vi "Read TCP FIFO.vi"(6 "Error In":errorcluster, 9 "Vessel.lvclass":refnum<class "Vessel.lvclass">) -> (0 "Error Out":errorcluster, 3 "Vessel.lvclass 2":refnum<class "Vessel.lvclass">)   [LabVIEW 2014, in "Vessel.lvclass"]
uses:
  Vessel.lvclass
  Vessel.lvclass/Vessel.ctl
  Supervisor/Supervisor.lvclass
panel:
  out "UDP GPS":string
  out "UDP APOS":string
  out "Camera Trigger Message":string
  out "UDP error out":errorcluster
  out "APOS NED":dbl[](array[numeric]) format="%#.3f"
  out "kPa":dbl=100000.0 format="%#.1f"
  in  "depth ring":u16(ring)=2 items=["Saiv", "DVL", "Digiquartz"]
  out "DVL":string
  out "MT_BITS":u8[](array[numeric])
  out "Pos_s":dbl[](array[numeric])
  out "Altitudes":dbl[](array[numeric])
  out "Telebuf":u8[](array[numeric])
  out "NAVI OK":string
  out "MT_DATA":sgl[](array[numeric])
  in  "alt off [m]":dbl=0.2
  out "dvl_m":dbl[](array[numeric])
  out "MRU out":dbl[](array[numeric])
  out "Signals out":dbl[](array[numeric]) format="%#.2f"
  # "10."
  # "20."
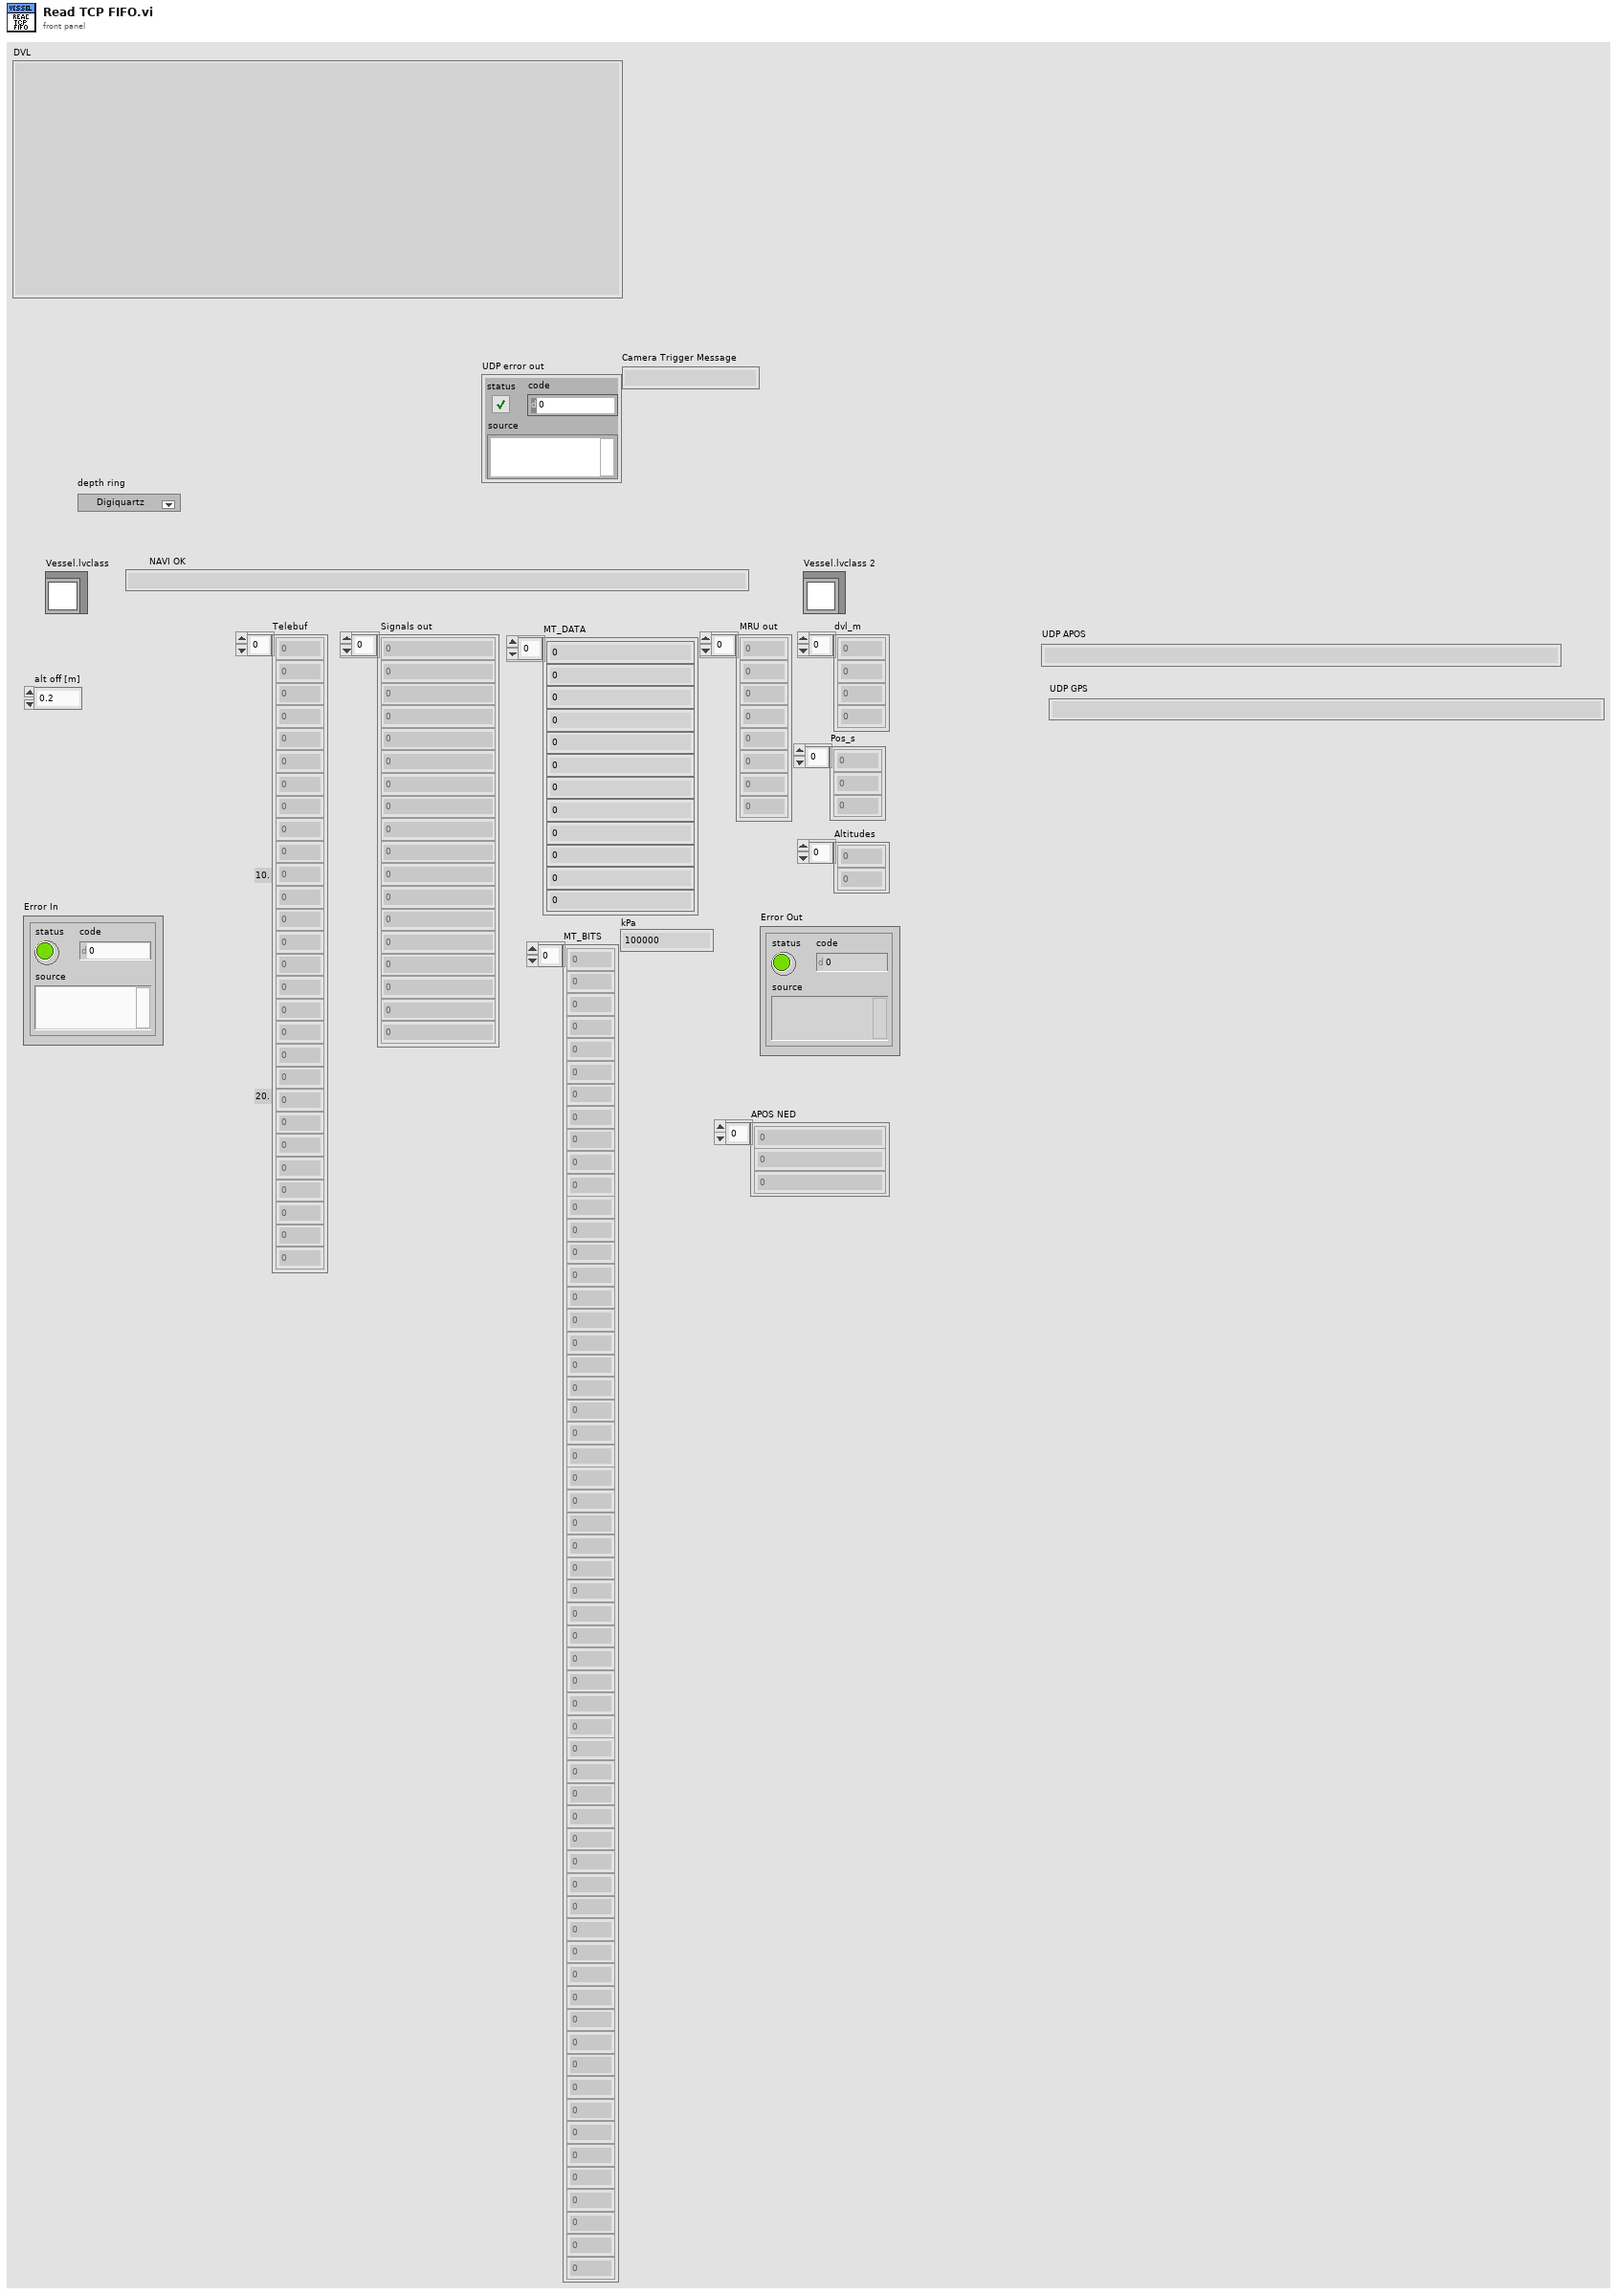
[diagram p1: front panel]
types:
  T1 = cluster{"Axis Translation":cluster{"X-Axis":dbl, "Y-Axis":dbl, "Z-Axis":dbl}, "Axis Rotation":cluster{"X-Axis":dbl, "Y-Axis":dbl, "Z-Axis":dbl}}
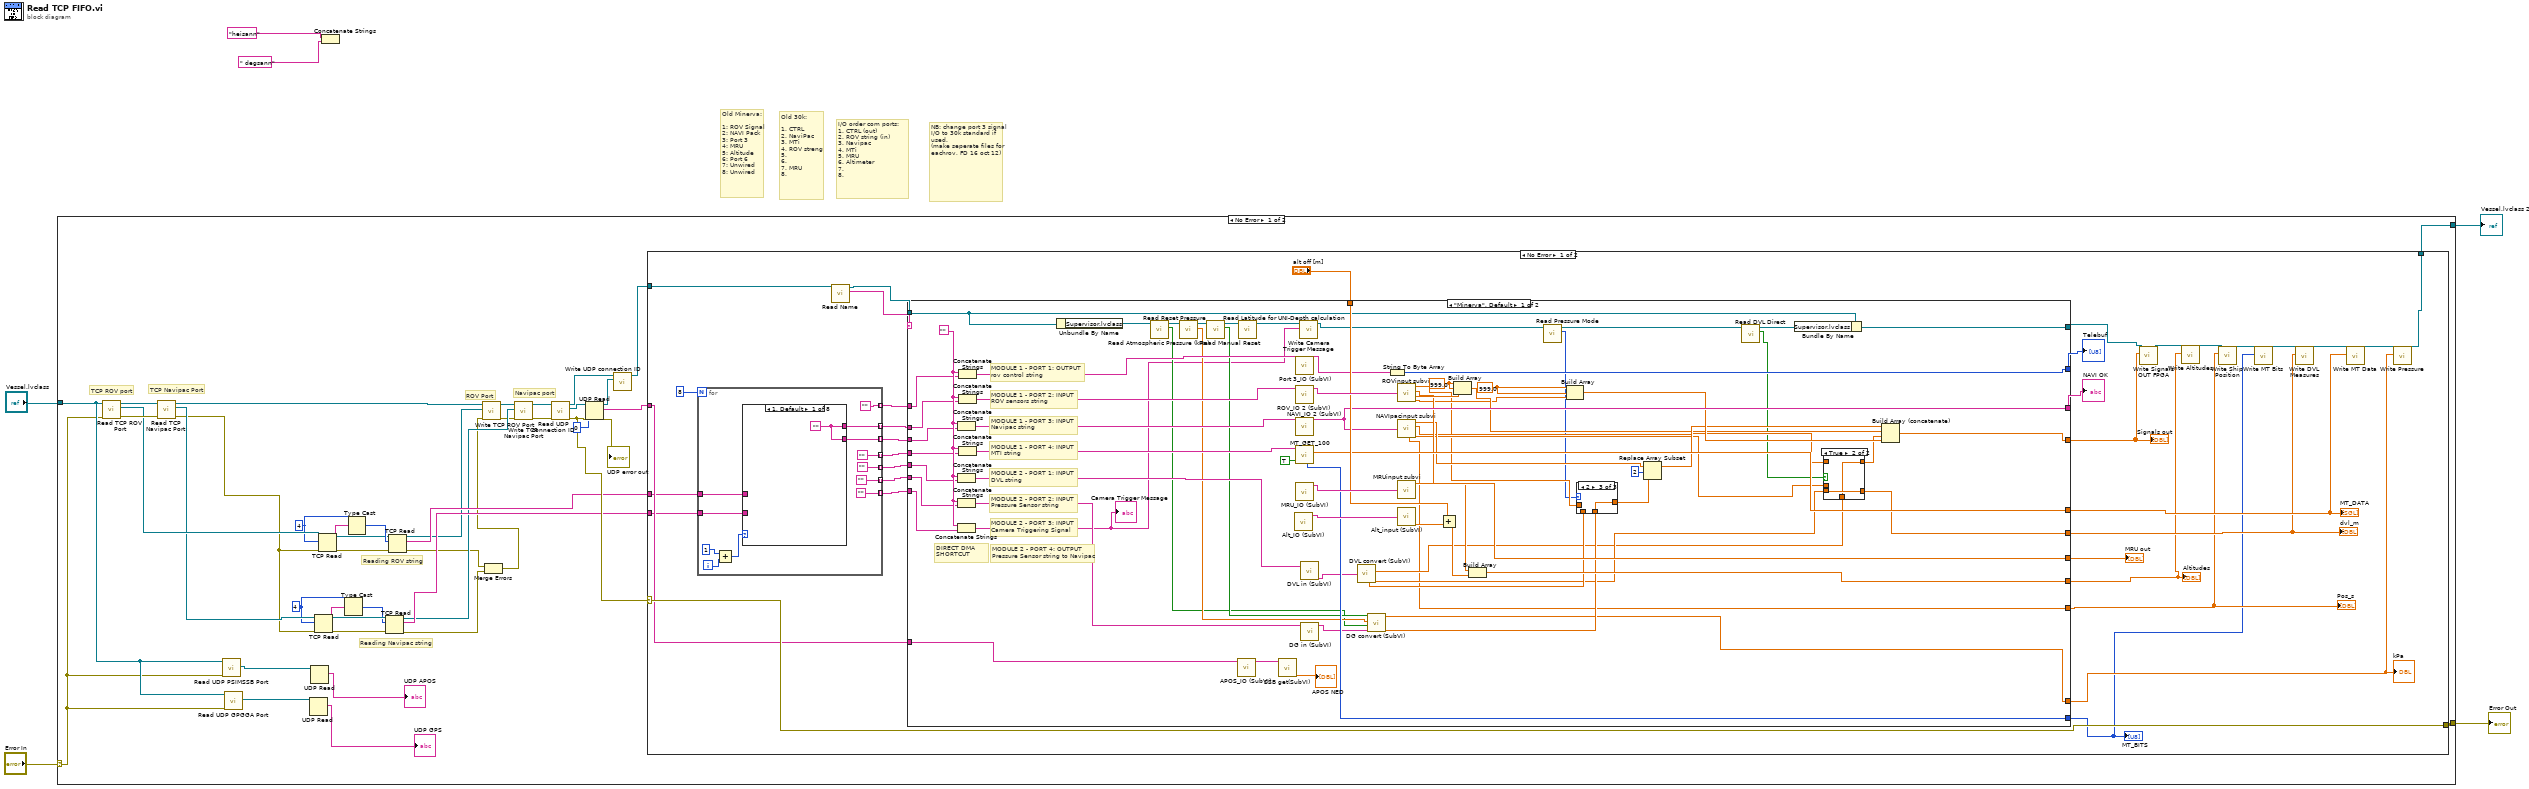
[diagram p0: block diagram]
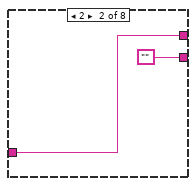
[diagram p2: hidden frame]
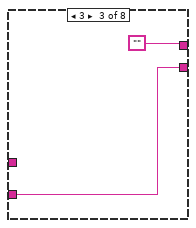
[diagram p3: hidden frame]
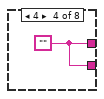
[diagram p4: hidden frame]
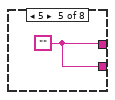
[diagram p5: hidden frame]
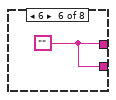
[diagram p6: hidden frame]
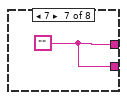
[diagram p7: hidden frame]
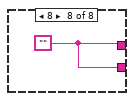
[diagram p8: hidden frame]
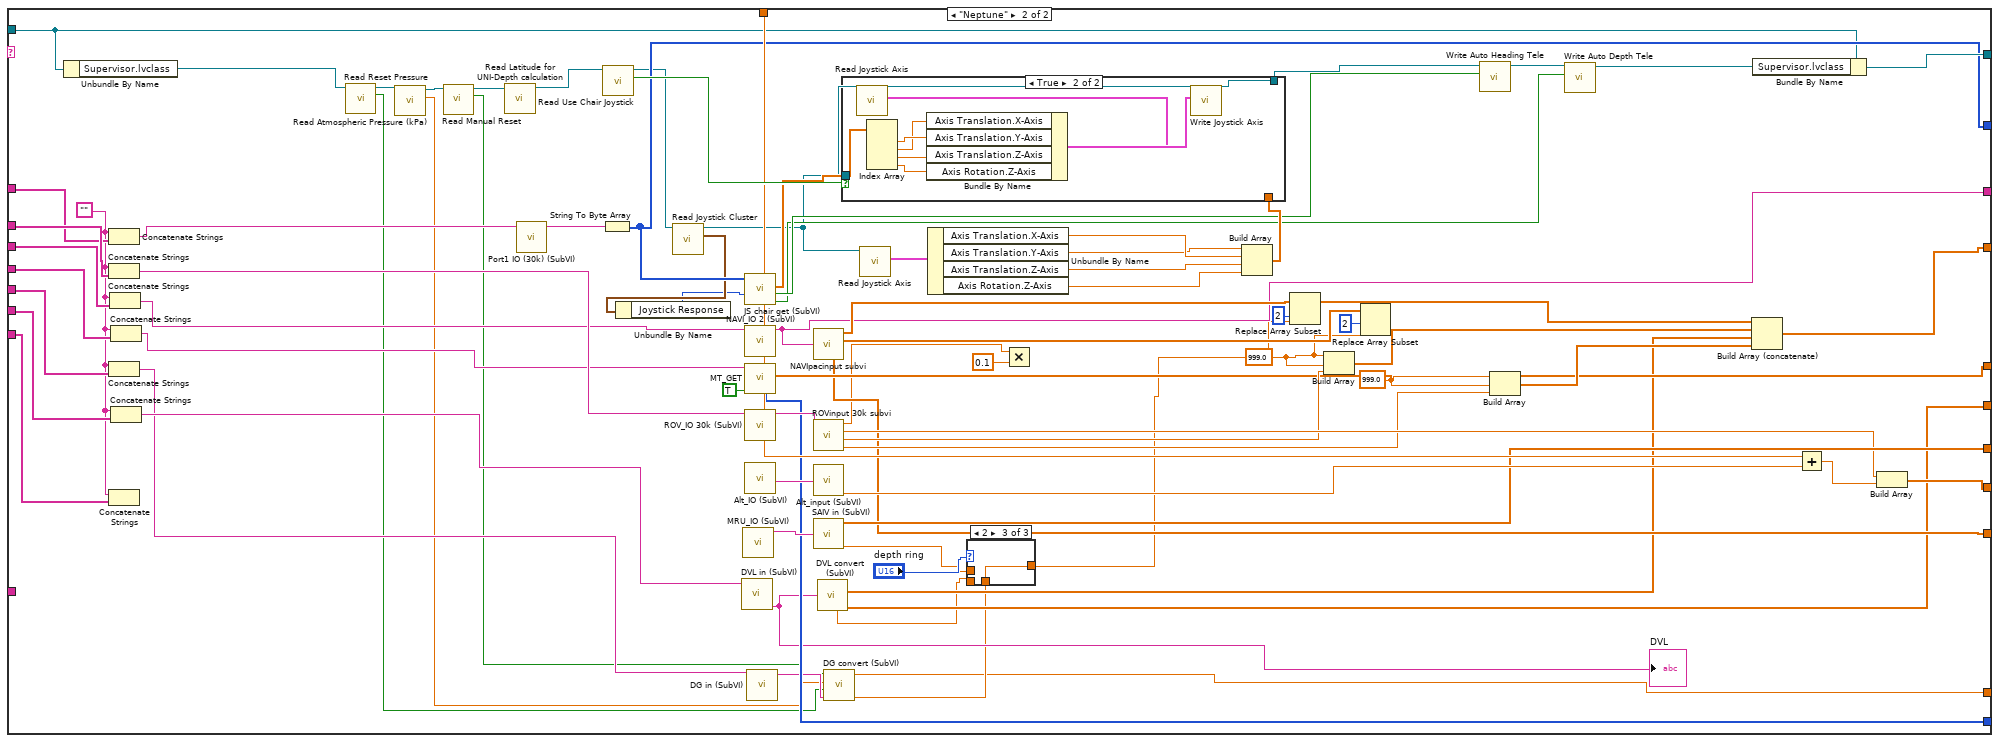
[diagram p12: hidden frame]
diagram:
  # "NB: change port 3 signal I/O to 30k standard if used. \n(make seperate files for eachrov, FD 16 oct 12)"
  # "I/O order com ports:\n1. CTRL (out)\n2. ROV string (in)\n3. Navipac\n4. MTi\n5. MRU\n6. Altimeter\n7. \n8."
  # "Old 30k:\n\n1. CTRL\n2. NaviPac\n3. MTi\n4. ROV streng\n5.\n6.\n7. MRU\n8."
  # "Old Minerva:\n\n1: ROV Signal\n2: NAVI Pack\n3: Port 3\n4: MRU\n5: Altitude \n6: Port 6\n7: Unwired\n8: Unwired"
  n1 = case shown="No Error" "Error In" {
    selector: "Error In" -> [w11 w282]
    tunnel: "Vessel.lvclass" -> [w12 w283]
    tunnel: [w49 w282] -> w4
    tunnel: [w48 w283] -> w3
    frame No Error {
      w19 = 4
      w20 = 4
      # "Reading ROV string"
      # "Reading Navipac string"
      # "Navipac port"
      # "ROV Port"
      # "TCP Navipac Port"
      # "TCP ROV port"
      n2 = call-dynamic "Read TCP ROV Port.vi"("error in (no error)"=w11, "Vessel in"=w12) -> ("error out"=w36:errorcluster, "TCP Network Connection Refnum"=w35:refnum<k5>, "Vessel out"=w37:refnum<class "Vessel.lvclass">)  [unwired: 7 in]
      n3 = call-dynamic "Read TCP Navipac Port.vi"("error in (no error)"=w36, "Vessel in"=w37) -> ("error out"=w33:errorcluster, "TCP Network Connection Refnum"=w34:refnum<k5>, "Vessel out"=w32:refnum<class "Vessel.lvclass">)  [unwired: 7 in]
      n4 = call-dynamic "Read UDP PSIMSSB Port.vi"("error in (no error)"=w11, "Vessel in"=w12) -> ("UDP Network Connection Refnum"=w10:refnum<k16>)  [unwired: 7 in, 2 out]
      n5 = call-dynamic "Read UDP GPGGA Port.vi"("error in (no error)"=w11, "Vessel in"=w12) -> ("UDP Network Connection Refnum"=w9:refnum<k16>)  [unwired: 7 in, 2 out]
      n6 = UDP Read(connection ID=w9) -> (data out=→"UDP GPS":string)  [unwired: 3 in, 4 out]
      n7 = UDP Read(connection ID=w10) -> (data out=→"UDP APOS":string)  [unwired: 3 in, 4 out]
      n8 = TCP Read(connection ID=w34, bytes to read=w20, error in (no error)=w33) -> (connection ID out=w24:refnum<k5>, data out=w22:string, error out=w23:errorcluster)  [unwired: 2 in]
      n9 = TCP Read(connection ID=w35, bytes to read=w19, error in (no error)=w33) -> (connection ID out=w15:refnum<k5>, data out=w17:string, error out=w16:errorcluster)  [unwired: 2 in]
      n10 = Type Cast(type=w20, x=w22) -> (*(type *) &x=w21:i32)
      n11 = Type Cast(type=w19, x=w17) -> (*(type *) &x=w18:i32)
      n12 = TCP Read(connection ID=w24, bytes to read=w21, error in (no error)=w23) -> (connection ID out=w28:refnum<k5>, data out=w38:string, error out=w14:errorcluster)  [unwired: 2 in]
      n13 = TCP Read(connection ID=w15, bytes to read=w18, error in (no error)=w16) -> (connection ID out=w29:refnum<k5>, data out=w39:string, error out=w13:errorcluster)  [unwired: 2 in]
      n14 = Merge Errors(w13, w14) -> (w27:errorcluster)
      n15 = call-dynamic "Write TCP ROV Port.vi"("error in (no error)"=w27, "TCP Network Connection Refnum"=w29, "Vessel in"=w32) -> ("error out"=w26:errorcluster, "Vessel out"=w31:refnum<class "Vessel.lvclass">)  [unwired: 7 in]
      n16 = call-dynamic "Write TCP Navipac Port.vi"("error in (no error)"=w26, "TCP Network Connection Refnum"=w28, "Vessel in"=w31) -> ("error out"=w25:errorcluster, "Vessel out"=w30:refnum<class "Vessel.lvclass">)  [unwired: 7 in]
      n17 = call-dynamic "Read UDP connection ID.vi"("error in (no error)"=w25, "Vessel in"=w30) -> ("error out"=w42:errorcluster, "UDP connection ID"=w47:refnum<k16>, "Vessel out"=w45:refnum<class "Vessel.lvclass">)  [unwired: 7 in]
      n18 = UDP Read(connection ID=w47, timeout ms (25000)=0, 8:w42) -> (data out=w46:string, error out=→"UDP error out":errorcluster, 3:w43:refnum<k16>)  [unwired: 1 in, 2 out]
      n19 = call-dynamic "Write UDP connection ID.vi"("UDP connection ID"=w43, "Vessel in"=w45) -> ("Vessel out"=w44:refnum<class "Vessel.lvclass">)  [unwired: 8 in, 1 out]
      n20 = case shown="No Error" w42 {
        selector: w42 -> [w79 w281]
        tunnel: [w79 w281] -> w49
        tunnel: w44 -> [w69 w280]
        tunnel: [w67 w280] -> w48
        tunnel: w46 -> [w68 _]
        tunnel: w39 -> [w52 _]
        tunnel: w38 -> [w51 _]
        frame No Error {
          n21 = for {
            N: 8 -> [_]
            tunnel: [""] -> w83 mode=indexing
            tunnel: [""] -> w80 mode=indexing
            tunnel: [""] -> w76 mode=indexing
            tunnel: [""] -> w75 mode=indexing
            tunnel: [""] -> w81 mode=indexing
            tunnel: w52 -> [w90]
            tunnel: w51 -> [w89]
            tunnel: [w85] -> w82 mode=indexing
            tunnel: [w84] -> w77 mode=indexing
            i -> [w87]
            n22 = Add(x=1, y=w87) -> (x+y=w86:i32)
            n23 = case shown="1, Default" w86 {
              tunnel: w90 -> [_ w98 _ _ _ _ _ _]
              tunnel: w89 -> [_ _ w100 _ _ _ _ _]
              tunnel: [w96 w98 "" w101 w102 w103 w104 w105] -> w85
              tunnel: [w96 "" w100 w101 w102 w103 w104 w105] -> w84
              frame 1, Default {
                w96 = ""
              }
              frame 2 {
              }
              frame 3 {
              }
              frame 4 {
                w101 = ""
              }
              frame 5 {
                w102 = ""
              }
              frame 6 {
                w103 = ""
              }
              frame 7 {
                w104 = ""
              }
              frame 8 {
                w105 = ""
              }
            }
          }
          n24 = call-dynamic "Read Name.vi"("Vessel in"=w69) -> ("Name"=w73:string, "Vessel out"=w74:refnum<class "Vessel.lvclass">)  [unwired: 8 in, 1 out]
          n25 = case shown="\"Minerva\", Default" w73 {
            tunnel: w83 -> [w173 w265]
            tunnel: w82 -> [w175 w264]
            tunnel: w81 -> [w176 w263]
            tunnel: [w152 w214] -> w59
            tunnel: w80 -> [w172 w262]
            tunnel: [w163 w213] -> w78
            tunnel: [w132 w204] -> w62
            tunnel: w77 -> [w174 w258]
            tunnel: w76 -> [w171 w257]
            tunnel: w74 -> [w148 w224]
            tunnel: [w147 w253] -> w60
            tunnel: w75 -> [w170 w239]
            tunnel: "alt off [m]" -> [w164 w237]
            tunnel: [w162 w236] -> w71
            tunnel: [w159 w212] -> w64
            tunnel: [w160 w235] -> w70
            tunnel: [w149 w225] -> w53
            tunnel: [w110 w211] -> w61
            tunnel: [w145 w223] -> w56
            tunnel: [w126 w194] -> w66
            tunnel: w68 -> [w123 _]
            frame "Minerva", Default {
              w154 = 999.0 ("element")
              w156 = 999.0 ("element")
              w177 = ""
              # "DIRECT DMA SHORTCUT"
              # "MODULE 2 - PORT 4: OUTPUT\nPressure Sensor string to Navipac"
              # "MODULE 2 - PORT 3: INPUT\nCamera Triggering Signal"
              # "MODULE 2 - PORT 2: INPUT\nPressure Sensor string"
              # "MODULE 2 - PORT 1: INPUT\nDVL string"
              # "MODULE 1 - PORT 4: INPUT\nMTI string"
              # "MODULE 1 - PORT 3: INPUT\nNavipac string"
              # "MODULE 1 - PORT 2: INPUT\nROV sensors string"
              # "MODULE 1 - PORT 1: OUTPUT\nrov control string"
              n26 = Concatenate Strings(w177, w174) -> (w158:string)
              n27 = Concatenate Strings(w177, w172) -> (w124:string)
              n28 = Concatenate Strings(w177, w171) -> (w138:string)
              n29 = Concatenate Strings(w177, w170) -> (w108:string)
              "Camera Trigger Message" <- w108
              n30 = Concatenate Strings(w177, w176) -> (w146:string)
              n31 = Concatenate Strings(w177, w175) -> (w125:string)
              n32 = Concatenate Strings(w177, w173) -> (w157:string)
              n33 = Unbundle By Name(w148) -> ("Supervisor.lvclass"=w115:refnum<class "Supervisor.lvclass">)
              n34 = call-dynamic "Read Reset Pressure.vi"("Supervisor in"=w115) -> ("Reset Pressure"=w112:bool, "Supervisor out"=w117:refnum<class "Supervisor.lvclass">)  [unwired: 8 in, 1 out]
              n35 = call-dynamic "Read Atmospheric Pressure (kPa).vi"("Supervisor in"=w117) -> ("Atmospheric Pressure (deciBar)"=w113:dbl, "Supervisor out"=w116:refnum<class "Supervisor.lvclass">)  [unwired: 8 in, 1 out]
              n36 = call-dynamic "Read Manual Reset.vi"("Supervisor in"=w116) -> ("Manual Reset"=w114:bool, "Supervisor out"=w107:refnum<class "Supervisor.lvclass">)  [unwired: 8 in, 1 out]
              n37 = call "APOS_IO (SubVI).vi"("GPS in"=w123) -> ("GPS OK"=w122:string)  [unwired: 9 in, 1 out]
              n38 = call-dynamic "Read Latitude for UNI-Depth calculation.vi"("Supervisor in"=w107) -> ("Supervisor out"=w106:refnum<class "Supervisor.lvclass">)  [unwired: 8 in, 2 out]
              n39 = call "SSB get(SubVI).vi"("String"=w122) -> ("APOS NED"=→"APOS NED":dbl[])  [unwired: 4 in, 1 out]
              n40 = call "Alt_IO (SubVI).vi"() -> ("Altimeter OK"=w167:string)  [unwired: 11 in]
              n41 = call "ROV_IO 2 (SubVI).vi"("ROV string"=w125) -> ("ROV OK"=w169:string)  [unwired: 10 in]
              n42 = call "NAVI_IO 2 (SubVI).vi"("NAVI string"=w158) -> ("NAVI OK"=w163:string)  [unwired: 10 in]
              n43 = call "MT_GET_100.vi"("Use checksum"=TRUE, "read buffer"=w157) -> ("MT_DATA"=w159:sgl[], "MT_BITS"=w145:u8[])  [unwired: 6 in, 2 out]
              n44 = call "Port 3_IO (SubVI).vi"("port 3 hex  string"=w146) -> ("port 3 OK"=w161:string)  [unwired: 10 in]
              n45 = call "MRU_IO (SubVI).vi"() -> ("MRU OK"=w166:string)  [unwired: 11 in]
              n46 = call-dynamic "Write Camera Trigger Message.vi"("Camera Trigger Message"=w108, "Supervisor in"=w106) -> ("Supervisor out"=w109:refnum<class "Supervisor.lvclass">)  [unwired: 8 in, 1 out]
              n47 = call "DVL in (SubVI).vi"("DVL string"=w124) -> ("DVL OK"=w143:string)  [unwired: 10 in]
              n48 = call "DG in (SubVI).vi"("DG string"=w138) -> ("DG OK"=w144:string)  [unwired: 10 in]
              n49 = call "DVL convert (SubVI).vi"("String"=w143) -> ("depth"=w136:dbl, "dvl alts"=w133:dbl[], "u_bt_dvl"=w128:dbl[])  [unwired: 1 in, 2 out]
              n50 = call "DG convert (SubVI).vi"("String"=w144, "Reset pressure"=w112, "atm kPa"=w113, "manual reset"=w114) -> ("depth"=w135:dbl, "Pressure (deciBAR = 10*kPASCAL)"=w126:dbl)  [unwired: 1 in, 1 out]
              n51 = String To Byte Array(string=w161) -> (unsigned byte array=w160:u8[])
              n52 = call "ROVinput subvi.vi"("String"=w169) -> ("depth"=w127:dbl, "altitude"=w151:dbl, "heading"=w155:dbl, "yaw rate"=w137:dbl)
              n53 = call "NAVIpacinput subvi.vi"("String"=w163) -> ("Pos_s"=w110:dbl[], "a_dvl"=w131:dbl[], "vb_dvl"=w130:dbl[], "NED_tp"=w142:dbl[])  [unwired: 2 out]
              n54 = call "MRUinput subvi.vi"("String"=w166) -> ("MRU out"=w162:dbl[])  [unwired: 3 in]
              n55 = call "Alt_input (SubVI).vi"("String"=w167) -> ("altitude"=w165:dbl)  [unwired: 3 in]
              n56 = Add(x=w164, y=w165) -> (x+y=w150:dbl)
              n57 = Build Array(w156, w156, w155) -> (w139:dbl[])
              n58 = Build Array(w151, w150) -> (w149:dbl[])
              n59 = call-dynamic "Read Pressure Mode.vi"("Supervisor in"=w109) -> ("Pressure Mode"=w118:i16, "Supervisor out"=w111:refnum<class "Supervisor.lvclass">)  [unwired: 8 in, 1 out]
              n60 = Build Array(w154, w154, w137) -> (w153:dbl[])
              n61 = case shown="2" w118 {
                tunnel: w136 -> [_ w183 _]
                tunnel: [w182 w183 w184] -> w134
                tunnel: w127 -> [w182 _ _]
                tunnel: w135 -> [_ _ w184]
                frame 0, Default {
                }
                frame 1 {
                }
                frame 2 {
                }
              }
              n62 = Replace Array Subset(array=w142, new element=w134, index=2) -> (w140:dbl[])
              n63 = call-dynamic "Read DVL Direct.vi"("Supervisor in"=w111) -> ("DVL Direct"=w119:bool, "Supervisor out"=w120:refnum<class "Supervisor.lvclass">)  [unwired: 8 in, 1 out]
              n64 = Bundle By Name(cluster=w148, "Supervisor.lvclass"=w120) -> (w147:refnum<class "Vessel.lvclass">)
              n65 = case shown="True" w119 {
                tunnel: w133 -> [_ w181]
                tunnel: [w179 w181] -> w132
                tunnel: w131 -> [w179 _]
                tunnel: w130 -> [w178 _]
                tunnel: [w178 w180] -> w129
                tunnel: w128 -> [_ w180]
                frame False {
                }
                frame True {
                }
              }
              n66 = Build Array (concatenate)(w140, w139, w129, w153) -> (w152:dbl[])
            }
            frame "Neptune" {
              w217 = 999.0 ("element")
              w206 = 999.0 ("element")
              w238 = ""
              n67 = Unbundle By Name(w224) -> ("Supervisor.lvclass"=w191:refnum<class "Supervisor.lvclass">)
              n68 = Concatenate Strings(w238, w263) -> (w256:string)
              n69 = Concatenate Strings(w238, w264) -> (w230:string)
              n70 = Concatenate Strings(w238, w262) -> (w196:string)
              n71 = Concatenate Strings(w238, w239) -> ()  [unwired: 1 out]
              n72 = Concatenate Strings(w238, w258) -> (w229:string)
              n73 = Concatenate Strings(w238, w265) -> (w228:string)
              n74 = Concatenate Strings(w238, w257) -> (w203:string)
              n75 = call-dynamic "Read Reset Pressure.vi"("Supervisor in"=w191) -> ("Reset Pressure"=w188:bool, "Supervisor out"=w193:refnum<class "Supervisor.lvclass">)  [unwired: 8 in, 1 out]
              n76 = call-dynamic "Read Atmospheric Pressure (kPa).vi"("Supervisor in"=w193) -> ("Atmospheric Pressure (deciBar)"=w189:dbl, "Supervisor out"=w192:refnum<class "Supervisor.lvclass">)  [unwired: 8 in, 1 out]
              n77 = call-dynamic "Read Manual Reset.vi"("Supervisor in"=w192) -> ("Manual Reset"=w190:bool, "Supervisor out"=w186:refnum<class "Supervisor.lvclass">)  [unwired: 8 in, 1 out]
              n78 = call-dynamic "Read Latitude for UNI-Depth calculation.vi"("Supervisor in"=w186) -> ("Supervisor out"=w185:refnum<class "Supervisor.lvclass">)  [unwired: 8 in, 2 out]
              n79 = call "Port1 IO (30k) (SubVI).vi"("port 3 hex  string"=w256) -> ("port 3 OK"=w255:string)  [unwired: 10 in]
              n80 = String To Byte Array(string=w255) -> (unsigned byte array=w235:u8[])
              n81 = call-dynamic "Read Use Chair Joystick.vi"("Supervisor in"=w185) -> ("Use Chair Joystick"=w254:bool, "Supervisor out"=w234:refnum<class "Supervisor.lvclass">)  [unwired: 8 in, 1 out]
              n82 = call-dynamic "Read Joystick Cluster.vi"("Supervisor in"=w234) -> ("Joystick Cluster"=w233:cluster{"Joystick Response":u16}, "Supervisor out"=w232:refnum<class "Supervisor.lvclass">)  [unwired: 8 in, 1 out]
              n83 = Unbundle By Name(w233) -> ("Joystick Response"=w231:u16)
              n84 = call "DVL in (SubVI).vi"("DVL string"=w203) -> ("DVL OK"=w202:string)  [unwired: 10 in]
              "DVL" <- w202
              n85 = call "MRU_IO (SubVI).vi"() -> ("MRU OK"=w261:string)  [unwired: 11 in]
              n86 = call "JS chair get (SubVI).vi"("JS resp"=w231, "Telebuf in"=w235) -> ("Auto Depth"=w242:bool, "Auto Heading"=w243:bool, "t_js_prc"=w246:dbl[])  [unwired: 6 in, 1 out]
              n87 = call "NAVI_IO 2 (SubVI).vi"("NAVI string"=w229) -> ("NAVI OK"=w213:string)  [unwired: 10 in]
              n88 = call "MT_GET.vi"("Use checksum"=TRUE, "read buffer"=w228) -> ("MT_DATA"=w212:sgl[], "MT_BITS"=w223:u8[])  [unwired: 6 in, 2 out]
              n89 = call "ROV_IO 30k (SubVI).vi"("ROV string"=w230) -> ("ROV OK"=w240:string)  [unwired: 10 in]
              n90 = call "Alt_IO (SubVI).vi"() -> ("Altimeter OK"=w260:string)  [unwired: 11 in]
              n91 = call "DG in (SubVI).vi"("DG string"=w196) -> ("DG OK"=w201:string)  [unwired: 10 in]
              n92 = call "NAVIpacinput subvi.vi"("String"=w213) -> ("Pos_s"=w211:dbl[], "vb_dvl"=w208:dbl[], "NED_tp"=w222:dbl[])  [unwired: 3 out]
              n93 = call "ROVinput 30k subvi.vi"("String"=w240) -> ("depth"=w209:dbl, "altitude"=w227:dbl, "heading"=w219:dbl, "yaw rate"=w216:dbl)
              n94 = call "Alt_input (SubVI).vi"("String"=w260) -> ("altitude"=w259:dbl)  [unwired: 3 in]
              n95 = call "SAIV in (SubVI).vi"("String"=w261) -> ("SAIV out"=w236:dbl[], "depth"=w197:dbl)  [unwired: 2 in]
              n96 = call "DVL convert (SubVI).vi"("String"=w202) -> ("depth"=w199:dbl, "dvl alts"=w204:dbl[], "u_bt_dvl"=w205:dbl[])  [unwired: 1 in, 2 out]
              n97 = call "DG convert (SubVI).vi"("String"=w201, "Reset pressure"=w188, "atm kPa"=w189, "manual reset"=w190) -> ("depth"=w195:dbl, "Pressure (deciBAR = 10*kPASCAL)"=w194:dbl)  [unwired: 1 in, 1 out]
              n98 = call-dynamic "Read Joystick Axis.vi"("Supervisor in"=w232) -> ("Joystick Axis"=w252:T1)  [unwired: 8 in, 2 out]
              n99 = Unbundle By Name(w252) -> ("Axis Translation.X-Axis"=w251:dbl, "Axis Translation.Y-Axis"=w250:dbl, "Axis Translation.Z-Axis"=w249:dbl, "Axis Rotation.Z-Axis"=w248:dbl)
              n100 = case shown="2" "depth ring" {
                tunnel: w199 -> [_ w267 _]
                tunnel: [w266 w267 w268] -> w198
                tunnel: w197 -> [w266 _ _]
                tunnel: w195 -> [_ _ w268]
                frame 0, Default {
                }
                frame 1 {
                }
                frame 2 {
                }
              }
              n101 = Multiply(x=w209, y=0.1) -> ()  [unwired: 1 out]
              n102 = Build Array(w250, w251, w249, w248) -> (w247:dbl[])
              n103 = case shown="True" w254 {
                tunnel: w246 -> [_ w276]
                tunnel: w232 -> [w269 w279]
                tunnel: [w269 w271] -> w245
                tunnel: w247 -> [_ _]
                frame False {
                }
                frame True {
                  n104 = call-dynamic "Read Joystick Axis.vi"("Supervisor in"=w279) -> ("Joystick Axis"=w270:T1, "Supervisor out"=w278:refnum<class "Supervisor.lvclass">)  [unwired: 8 in, 1 out]
                  n105 = Index Array(array=w276) -> (element #1=w275:dbl, element #2=w274:dbl, element #3=w273:dbl, element #4=w272:dbl)  [unwired: 4 in]
                  n106 = Bundle By Name(cluster=w270, "Axis Translation.X-Axis"=w274, "Axis Translation.Y-Axis"=w275, "Axis Translation.Z-Axis"=w273, "Axis Rotation.Z-Axis"=w272) -> (w277:T1)
                  n107 = call-dynamic "Write Joystick Axis.vi"("Joystick Axis"=w277, "Supervisor in"=w278) -> ("Supervisor out"=w271:refnum<class "Supervisor.lvclass">)  [unwired: 8 in, 1 out]
                }
              }
              n108 = Replace Array Subset(array=w222, new element=w198, index=2) -> (w220:dbl[])
              n109 = Build Array(w206, w206, w219) -> (w218:dbl[])
              n110 = Replace Array Subset(array=w208, new element=w206, index=2) -> ()  [unwired: 1 out]
              n111 = call-dynamic "Write Auto Heading Tele.vi"("Auto Heading Tele"=w243, "Supervisor in"=w245) -> ("Supervisor out"=w244:refnum<class "Supervisor.lvclass">)  [unwired: 8 in, 1 out]
              n112 = Build Array(w217, w217, w216) -> (w215:dbl[])
              n113 = call-dynamic "Write Auto Depth Tele.vi"("Auto Depth Tele"=w242, "Supervisor in"=w244) -> ("Supervisor out"=w187:refnum<class "Supervisor.lvclass">)  [unwired: 8 in, 1 out]
              n114 = Build Array (concatenate)(w220, w218, w205, w215) -> (w214:dbl[])
              n115 = Bundle By Name(cluster=w224, "Supervisor.lvclass"=w187) -> (w253:refnum<class "Vessel.lvclass">)
              n116 = Add(x=w237, y=w259) -> (x+y=w226:dbl)
              n117 = Build Array(w227, w226) -> (w225:dbl[])
            }
          }
          "Signals out" <- w59
          "dvl_m" <- w62
          "NAVI OK" <- w78
          "MRU out" <- w71
          "MT_DATA" <- w64
          "Telebuf" <- w70
          "Altitudes" <- w53
          "Pos_s" <- w61
          "MT_BITS" <- w56
          "kPa" <- w66
          n118 = call-dynamic "Write Signals OUT FPGA.vi"("Signals OUT"=w59, "Vessel in"=w60) -> ("Vessel out"=w55:refnum<class "Vessel.lvclass">)  [unwired: 8 in, 1 out]
          n119 = call-dynamic "Write Altitudes.vi"("Altitudes"=w53, "Vessel in"=w55) -> ("Vessel out"=w54:refnum<class "Vessel.lvclass">)  [unwired: 8 in, 1 out]
          n120 = call-dynamic "Write Ship Position.vi"("Ship Position"=w61, "Vessel in"=w54) -> ("Vessel out"=w57:refnum<class "Vessel.lvclass">)  [unwired: 8 in, 1 out]
          n121 = call-dynamic "Write MT Bits.vi"("MT Bits"=w56, "Vessel in"=w57) -> ("Vessel out"=w58:refnum<class "Vessel.lvclass">)  [unwired: 8 in, 1 out]
          n122 = call-dynamic "Write DVL Measures.vi"("DVL Measures"=w62, "Vessel in"=w58) -> ("Vessel out"=w63:refnum<class "Vessel.lvclass">)  [unwired: 8 in, 1 out]
          n123 = call-dynamic "Write MT Data.vi"("MT Data"=w64, "Vessel in"=w63) -> ("Vessel out"=w65:refnum<class "Vessel.lvclass">)  [unwired: 8 in, 1 out]
          n124 = call-dynamic "Write Pressure.vi"("Pressure"=w66, "Vessel in"=w65) -> ("Vessel out"=w67:refnum<class "Vessel.lvclass">)  [unwired: 8 in, 1 out]
        }
        frame Error {
        }
      }
    }
    frame Error {
    }
  }
  "Vessel.lvclass 2" <- w3
  "Error Out" <- w4
  n125 = Concatenate Strings("heisann", " degsann") -> ()  [unwired: 1 out]
